vi "JSON Tree Base Type to String.vi"(8 "error in (no error)":errorcluster, 11 "JSON Tree Base Type":variant) -> (0 "error out":errorcluster, 2 "JSON Tree Base Type String":string)   [LabVIEW 2011, in "i3-json.lvlib"]
doc: "Use this template to build a VI to use as a subVI."
uses:
  i3-json.lvlib
  JSON Types/JSON Type.ctl
  JSON Types/JSON Variant Attribute.ctl
  JSON Types/JSON Compatible Type.ctl
  Generation Error.ctl
  JSON Types/JSON Value String.ctl
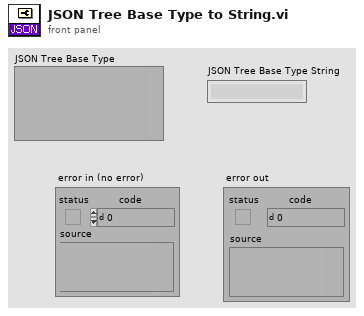
[diagram p1: front panel]
types:
  T1 = typedef "i3-json.lvlib/JSON Type.ctl" = enum8{"JSON Compatible", "JSON Array", "JSON Object", "JSON Null", "Double", "String", "Boolean", "Unknown"}
  T2 = typedef "i3-json.lvlib/JSON Variant Attribute.ctl" = string
  T3 = typedef "i3-json.lvlib/JSON Compatible Type.ctl" = enum16{"1D Double Array", "1D String Array", "1D Boolean Array", "Unknown"}
  T4 = typedef "i3-json.lvlib/Generation Error.ctl" = string
  T5 = typedef "i3-json.lvlib/JSON Value String.ctl" = string
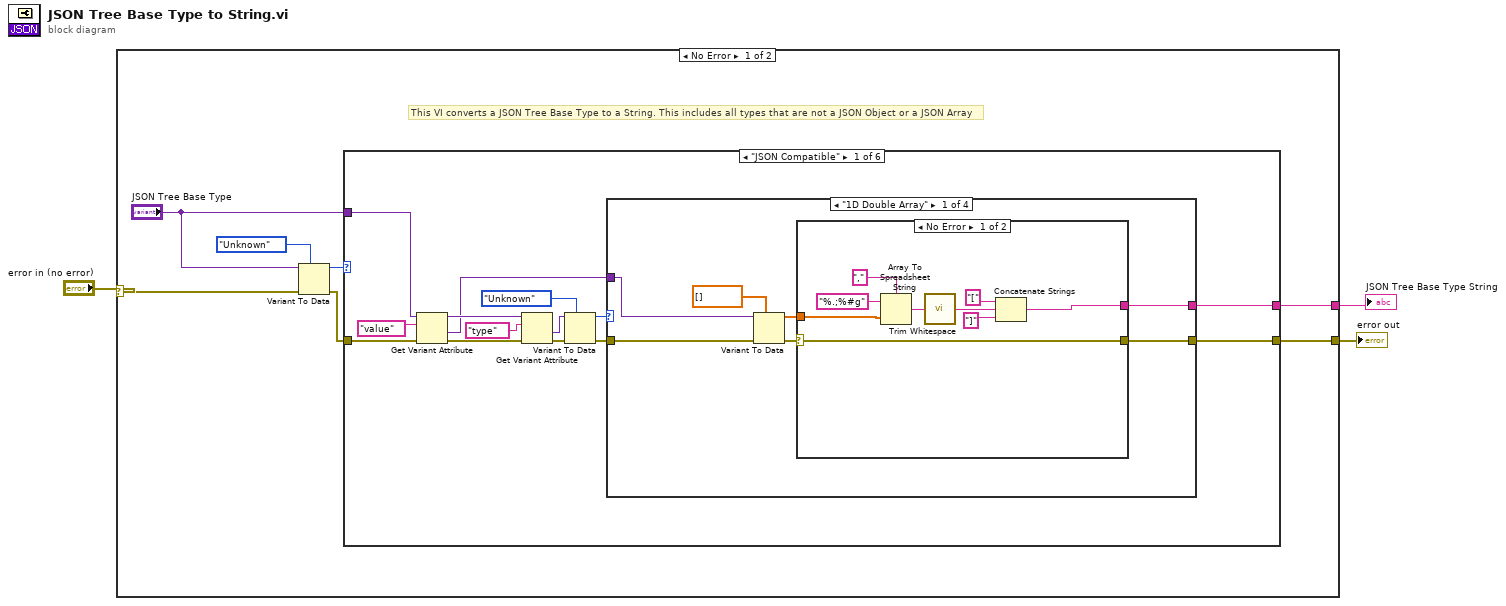
[diagram p0: block diagram]
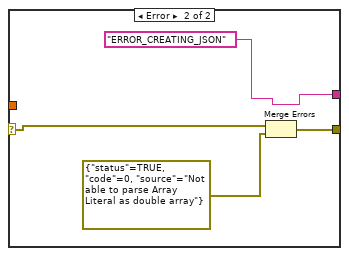
[diagram p2: hidden frame]
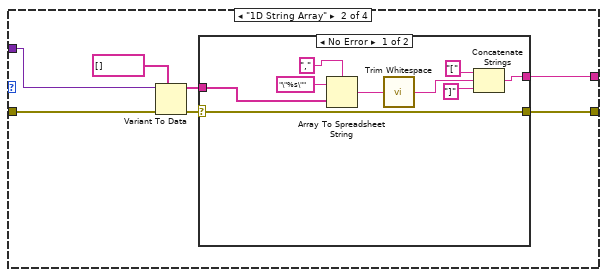
[diagram p3: hidden frame]
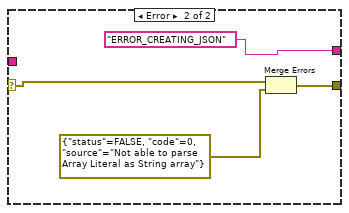
[diagram p4: hidden frame]
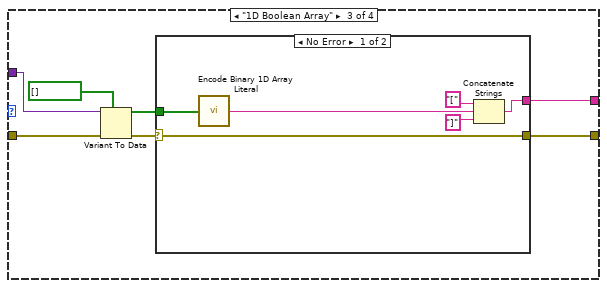
[diagram p5: hidden frame]
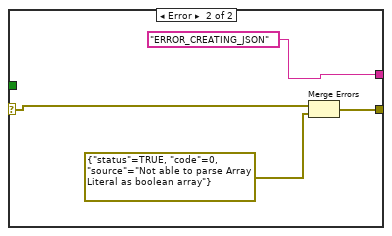
[diagram p6: hidden frame]
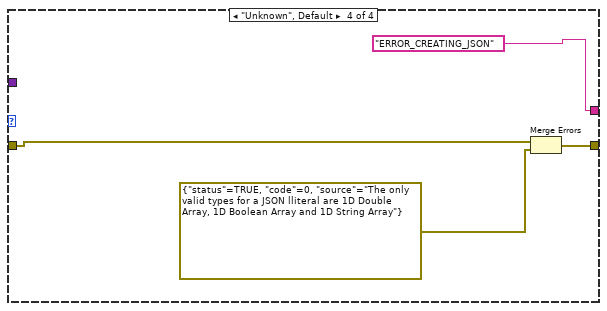
[diagram p7: hidden frame]
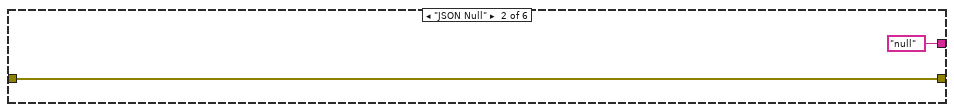
[diagram p8: hidden frame]
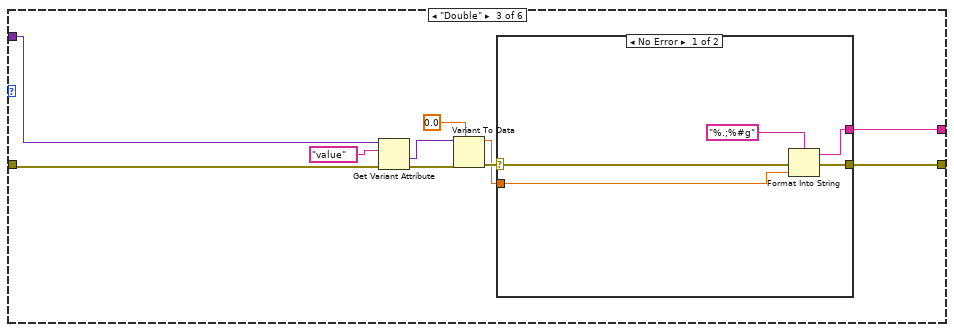
[diagram p9: hidden frame]
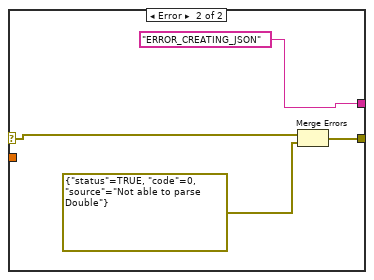
[diagram p10: hidden frame]
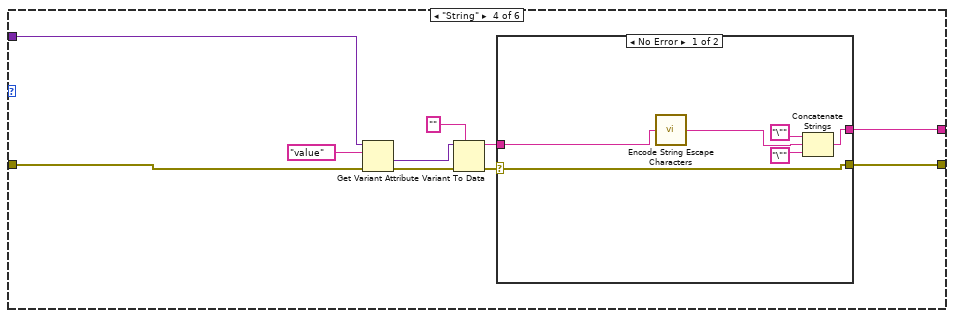
[diagram p11: hidden frame]
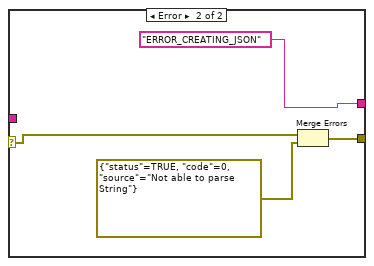
[diagram p12: hidden frame]
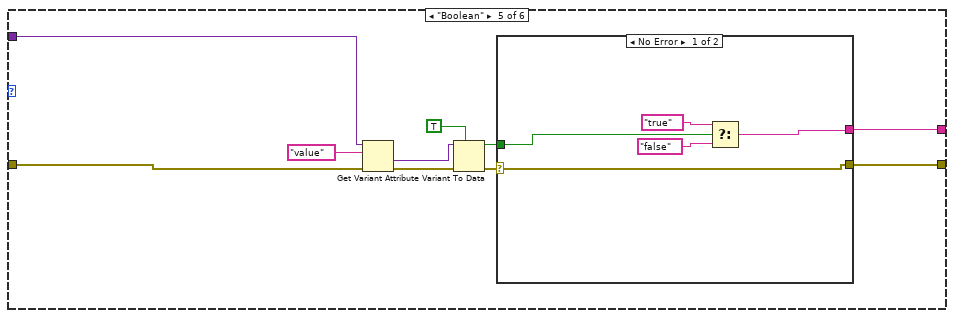
[diagram p13: hidden frame]
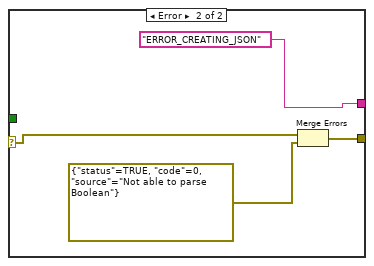
[diagram p14: hidden frame]
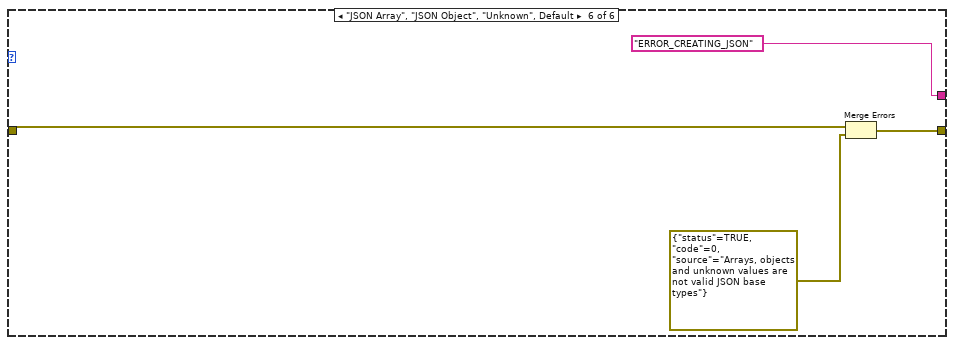
[diagram p15: hidden frame]
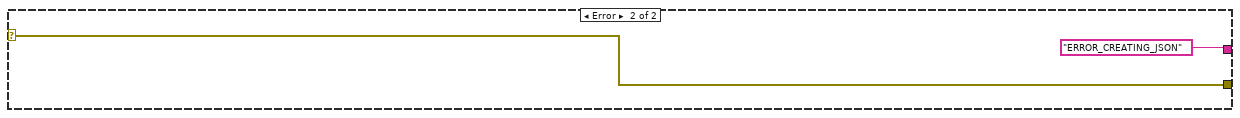
[diagram p16: hidden frame]
diagram:
  n1 = case shown="No Error" "error in (no error)" {
    selector: "error in (no error)" -> [w10 w151]
    tunnel: [w7 w151] -> w2
    tunnel: [w4 T4 "ERROR_CREATING_JSON" ("Generating Error")] -> w1
    frame No Error {
      # "This VI converts a JSON Tree Base Type to a String. This includes all types that are not a JSON Object or a JSON Array"
      n2 = Variant To Data(error in=w10, type=JSON_Type."Unknown" ("JSON Type"), Variant="JSON Tree Base Type") -> (data=w8:T1, error out=w6:errorcluster)
      n3 = case shown="\"JSON Compatible\"" w8 {
        tunnel: [w14 T5 "null" ("JSON Value String") w93 w109 w129 T4 "ERROR_CREATING_JSON" ("Generating Error")] -> w4
        tunnel: [w13 w86 w94 w110 w130 w149] -> w7
        tunnel: w6 -> [w12 w86 w88 w107 w127 w147]
        tunnel: "JSON Tree Base Type" -> [w11 _ w92 w108 w128 _]
        frame "JSON Compatible" {
          n4 = Get Variant Attribute(Variant=w11, name=T2 "value" ("JSON Variant Attribute"), error in=w12) -> (duplicate Variant=w18:variant, value=w15:variant, error out=w17:errorcluster)  [unwired: 1 in, 1 out]
          n5 = Get Variant Attribute(Variant=w18, name=T2 "type" ("JSON Variant Attribute"), error in=w17) -> (value=w23:variant, error out=w21:errorcluster)  [unwired: 1 in, 2 out]
          n6 = Variant To Data(error in=w21, type=JSON_Compatible_Type."Unknown" ("JSON Compatible Type"), Variant=w23) -> (data=w20:T3, error out=w19:errorcluster)
          n7 = case shown="\"1D Double Array\"" w20 {
            tunnel: w19 -> [w30 w47 w69 w83]
            tunnel: [w27 w45 w66 w85] -> w13
            tunnel: w15 -> [w31 w48 w68 _]
            tunnel: [w25 w46 w65 T4 "ERROR_CREATING_JSON" ("Generating Error")] -> w14
            frame "1D Double Array" {
              n8 = Variant To Data(error in=w30, type=dbl[] [], Variant=w31) -> (data=w26:dbl[], error out=w28:errorcluster)
              n9 = case shown="No Error" w28 {
                selector: w28 -> [w33 w42]
                tunnel: [w33 w44] -> w27
                tunnel: w26 -> [w40 _]
                tunnel: [w34 T4 "ERROR_CREATING_JSON" ("Generating Error")] -> w25
                frame No Error {
                  n10 = Array To Spreadsheet String(delimiter (Tab)=",", array=w40, 3:"%.;%#g" ("format string")) -> (spreadsheet string=w36:string)
                  n11 = call <vilib>:"Trim Whitespace.vi"("string"=w36) -> ("trimmed string"=w32:string)  [unwired: 1 in]
                  n12 = Concatenate Strings("[" ("string"), w32, "]" ("string")) -> (w34:string)
                }
                frame Error {
                  n13 = Merge Errors(w42, errorcluster {"status"=TRUE, "code"=0, "source"="Not able to parse Array Literal as double array"} ("error in")) -> (w44:errorcluster)
                }
              }
            }
            frame "1D String Array" {
              n14 = Variant To Data(error in=w47, type=string[] [], Variant=w48) -> (data=w49:string[], error out=w50:errorcluster)
              n15 = case shown="No Error" w50 {
                selector: w50 -> [w53 w62]
                tunnel: [w53 w64] -> w45
                tunnel: w49 -> [w60 _]
                tunnel: [w54 T4 "ERROR_CREATING_JSON" ("Generating Error")] -> w46
                frame No Error {
                  n16 = Array To Spreadsheet String(delimiter (Tab)=",", array=w60, 3:"\"%s\"" ("format string")) -> (spreadsheet string=w56:string)
                  n17 = call <vilib>:"Trim Whitespace.vi"("string"=w56) -> ("trimmed string"=w52:string)  [unwired: 1 in]
                  n18 = Concatenate Strings("[" ("string"), w52, "]" ("string")) -> (w54:string)
                }
                frame Error {
                  n19 = Merge Errors(w62, errorcluster {"status"=FALSE, "code"=0, "source"="Not able to parse Array Literal as String array"} ("error in")) -> (w64:errorcluster)
                }
              }
            }
            frame "1D Boolean Array" {
              n20 = Variant To Data(error in=w69, type=bool[] [], Variant=w68) -> (data=w70:bool[], error out=w67:errorcluster)
              n21 = case shown="No Error" w67 {
                selector: w67 -> [w74 w79]
                tunnel: [w74 w81] -> w66
                tunnel: w70 -> [w72 _]
                tunnel: [w75 T4 "ERROR_CREATING_JSON" ("Generating Error")] -> w65
                frame No Error {
                  n22 = call "Encode Binary 1D Array Literal.vi"("Array"=w72) -> ("string"=w73:string)
                  n23 = Concatenate Strings("[" ("string"), w73, "]" ("string")) -> (w75:string)
                }
                frame Error {
                  n24 = Merge Errors(w79, errorcluster {"status"=TRUE, "code"=0, "source"="Not able to parse Array Literal as boolean array"} ("error in")) -> (w81:errorcluster)
                }
              }
            }
            frame "Unknown", Default {
              n25 = Merge Errors(w83, errorcluster {"status"=TRUE, "code"=0, "source"="The only valid types for a JSON lliteral are 1D Double Array, 1D Boolean Array and 1D String Array"} ("error out")) -> (w85:errorcluster)
            }
          }
        }
        frame "JSON Null" {
        }
        frame "Double" {
          n26 = Get Variant Attribute(Variant=w92, name=T2 "value" ("JSON Variant Attribute"), error in=w88) -> (value=w91:variant, error out=w90:errorcluster)  [unwired: 1 in, 2 out]
          n27 = Variant To Data(error in=w90, type=0.0, Variant=w91) -> (data=w95:dbl, error out=w96:errorcluster)
          n28 = case shown="No Error" w96 {
            selector: w96 -> [w102 w104]
            tunnel: w95 -> [w101 _]
            tunnel: [w98 w106] -> w94
            tunnel: [w99 T4 "ERROR_CREATING_JSON" ("Generating Error")] -> w93
            frame No Error {
              n29 = Format Into String(format string="%.;%#g", error in=w102, w101) -> (resulting string=w99:string, error out=w98:errorcluster)  [unwired: 1 in]
            }
            frame Error {
              n30 = Merge Errors(w104, errorcluster {"status"=TRUE, "code"=0, "source"="Not able to parse Double"} ("error in")) -> (w106:errorcluster)
            }
          }
        }
        frame "String" {
          n31 = Get Variant Attribute(Variant=w108, name=T2 "value" ("JSON Variant Attribute"), error in=w107) -> (value=w114:variant, error out=w112:errorcluster)  [unwired: 1 in, 2 out]
          n32 = Variant To Data(error in=w112, type="", Variant=w114) -> (data=w116:string, error out=w115:errorcluster)
          n33 = case shown="No Error" w115 {
            selector: w115 -> [w122 w124]
            tunnel: w116 -> [w118 _]
            tunnel: [w122 w126] -> w110
            tunnel: [w121 T4 "ERROR_CREATING_JSON" ("Generating Error")] -> w109
            frame No Error {
              n34 = call "Encode String Escape Characters.vi"("unescaped string in"=w118) -> ("escaped string out"=w117:string)
              n35 = Concatenate Strings("\"" ("string"), w117, "\"" ("string")) -> (w121:string)
            }
            frame Error {
              n36 = Merge Errors(w124, errorcluster {"status"=TRUE, "code"=0, "source"="Not able to parse String"} ("error in")) -> (w126:errorcluster)
            }
          }
        }
        frame "Boolean" {
          n37 = Get Variant Attribute(Variant=w128, name=T2 "value" ("JSON Variant Attribute"), error in=w127) -> (value=w134:variant, error out=w133:errorcluster)  [unwired: 1 in, 2 out]
          n38 = Variant To Data(error in=w133, type=TRUE, Variant=w134) -> (data=w136:bool, error out=w135:errorcluster)
          n39 = case shown="No Error" w135 {
            selector: w135 -> [w141 w143]
            tunnel: w136 -> [w140 _]
            tunnel: [w141 w145] -> w130
            tunnel: [w137 T4 "ERROR_CREATING_JSON" ("Generating Error")] -> w129
            frame No Error {
              n40 = Select(t=T5 "true" ("JSON Value String"), s=w140, f=T5 "false" ("JSON Value String")) -> (s? t:f=w137:T5)
            }
            frame Error {
              n41 = Merge Errors(w143, errorcluster {"status"=TRUE, "code"=0, "source"="Not able to parse Boolean"} ("error in")) -> (w145:errorcluster)
            }
          }
        }
        frame "JSON Array", "JSON Object", "Unknown", Default {
          n42 = Merge Errors(w147, errorcluster {"status"=TRUE, "code"=0, "source"="Arrays, objects and unknown values are not valid JSON base types"} ("error in")) -> (w149:errorcluster)
        }
      }
    }
    frame Error {
    }
  }
  "error out" <- w2
  "JSON Tree Base Type String" <- w1
